vi "Temp_set_statemachine.vi"() -> ()   [LabVIEW 2022 SP3]
uses:
  set_temp_and_time_enum.ctl
  Command_buttons.ctl
  ctl_timer_fgv_states_enum.ctl
  Written_command.ctl
  Prog_time_control.ctl
panel:
  in  "stop":bool
  in  "Temp1 reached? 2":bool
  in  "Temp1 reached?":bool
  out "Written command":T1
  in  "Temperature-time\nprogram":T2
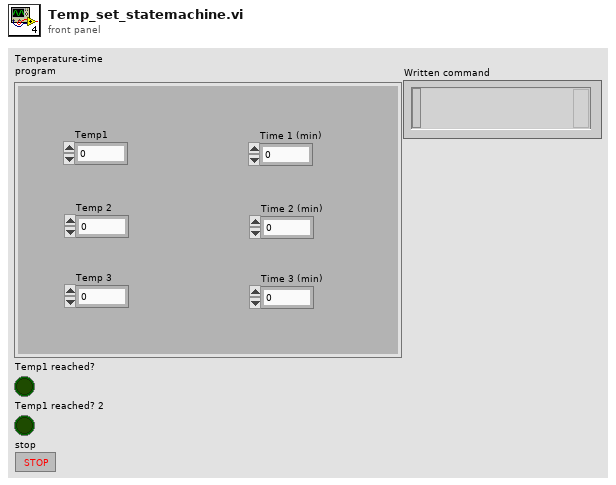
[diagram p1: front panel]
types:
  T1 = typedef "Written_command.ctl" = string
  T2 = typedef "Prog_time_control.ctl" = cluster{"Temp1":dbl, "Temp 2":dbl, "Temp 3":dbl, "Time 1 (min)":dbl, "Time 2 (min)":dbl, "Time 3 (min)":dbl}
  T3 = typedef "set_temp_and_time_enum.ctl" = enum16{"Init", "Set temp1", "Temp1 reached", "Set temp 2", "Temp2 reached", "Set temp 3", "Temp3 reached", "End"}
  T4 = typedef "ctl_timer_fgv_states_enum.ctl" = enum16{"RESET", "GET"}
  T5 = typedef "Command_buttons.ctl" = enum32{"P0", "P1", "F?", "S?", "Sn", "UC", "UF"}
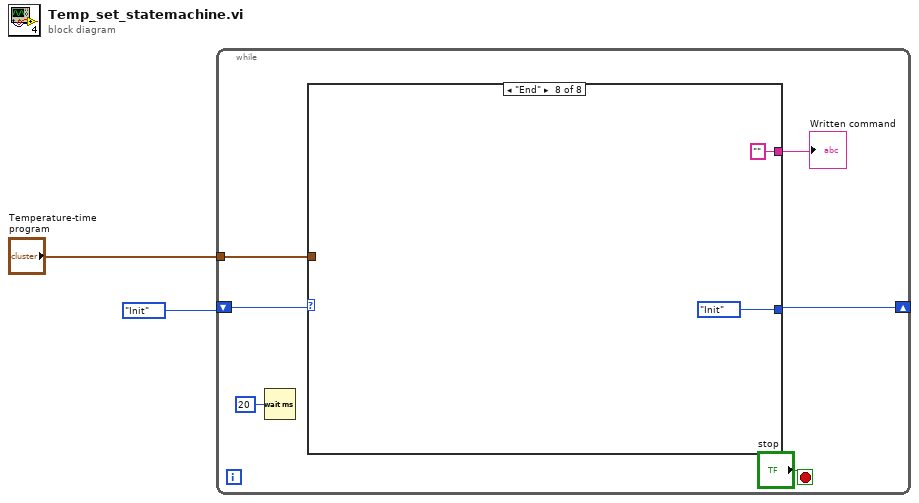
[diagram p0: block diagram]
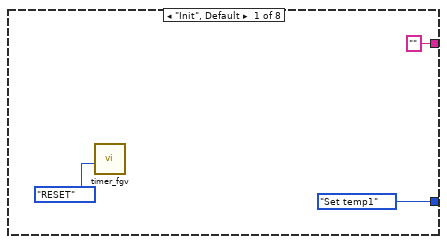
[diagram p2: hidden frame]
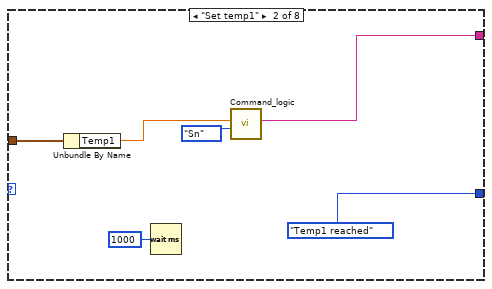
[diagram p3: hidden frame]
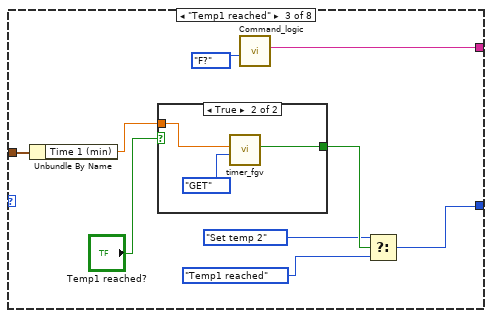
[diagram p4: hidden frame]
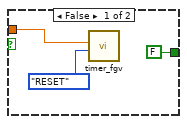
[diagram p5: hidden frame]
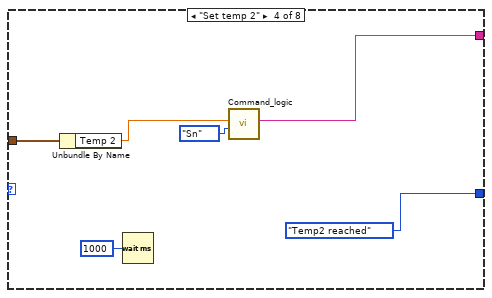
[diagram p6: hidden frame]
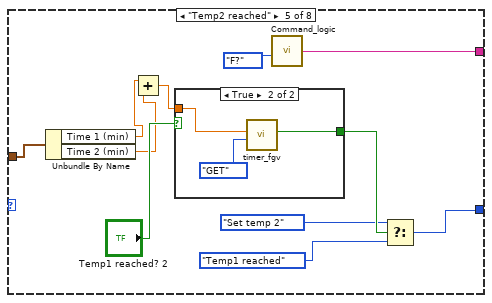
[diagram p7: hidden frame]
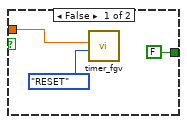
[diagram p8: hidden frame]
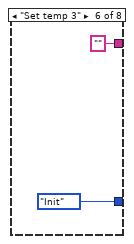
[diagram p9: hidden frame]
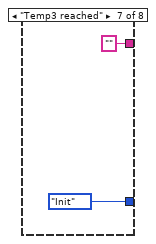
[diagram p10: hidden frame]
diagram:
  n1 = while {
    tunnel: "Temperature-time\nprogram" -> [w8]
    shift-right: [w7] -> _
    shift-left: set_temp_and_time_enum."Init" ("Enum") -> [w6]
    stop <- "stop" stop-if-true
    n2 = Wait (ms)(milliseconds to wait=u32 20) -> ()  [unwired: 1 out]
    n3 = case shown="\"End\"" w6 {
      tunnel: w8 -> [_ w16 w25 w37 w45 _ _ _]
      tunnel: [T1 "" ("Written command") w14 w18 w35 w40 T1 "" ("Written command") T1 "" ("Written command") T1 "" ("Written command")] -> w3
      tunnel: [set_temp_and_time_enum."Set temp1" ("Enum") set_temp_and_time_enum."Temp1 reached" ("Enum") w20 set_temp_and_time_enum."Temp2 reached" ("Enum") w39 set_temp_and_time_enum."Init" ("Enum") set_temp_and_time_enum."Init" ("Enum") set_temp_and_time_enum."Init" ("Enum")] -> w7
      frame "Init", Default {
        n4 = call "timer_fgv.vi"("Operation"=ctl_timer_fgv_states_enum."RESET") -> ()  [unwired: 10 in, 1 out]
      }
      frame "Set temp1" {
        n5 = Unbundle By Name(w16) -> ("Temp1"=w15:dbl)
        n6 = Wait (ms)(milliseconds to wait=u32 1000) -> ()  [unwired: 1 out]
        n7 = call "Command_logic.vi"("Command Radio Buttons"=Command_buttons."Sn", "Temperature\nto set"=w15) -> ("Written command"=w14:T1)  [unwired: 9 in]
      }
      frame "Temp1 reached" {
        n8 = Unbundle By Name(w25) -> ("Time 1 (min)"=w24:dbl)
        n9 = case shown="True" "Temp1 reached?" {
          tunnel: w24 -> [w28 w32]
          tunnel: [FALSE ("TIme passed?") w30] -> w23
          frame False {
            n10 = call "timer_fgv.vi"("Operation"=ctl_timer_fgv_states_enum."RESET", "TImer"=w28) -> ()  [unwired: 9 in, 1 out]
          }
          frame True {
            n11 = call "timer_fgv.vi"("Operation"=ctl_timer_fgv_states_enum."GET", "TImer"=w32) -> ("TIme passed?"=w30:bool)  [unwired: 9 in]
          }
        }
        n12 = call "Command_logic.vi"("Command Radio Buttons"=Command_buttons."F?") -> ("Written command"=w18:T1)  [unwired: 10 in]
        n13 = Select(t=set_temp_and_time_enum."Set temp 2" ("Enum"), s=w23, f=set_temp_and_time_enum."Temp1 reached" ("Enum")) -> (s? t:f=w20:T3)
      }
      frame "Set temp 2" {
        n14 = Unbundle By Name(w37) -> ("Temp 2"=w36:dbl)
        n15 = Wait (ms)(milliseconds to wait=u32 1000) -> ()  [unwired: 1 out]
        n16 = call "Command_logic.vi"("Command Radio Buttons"=Command_buttons."Sn", "Temperature\nto set"=w36) -> ("Written command"=w35:T1)  [unwired: 9 in]
      }
      frame "Temp2 reached" {
        n17 = Unbundle By Name(w45) -> ("Time 1 (min)"=w43:dbl, "Time 2 (min)"=w42:dbl)
        n18 = Add(x=w43, y=w42) -> (x+y=w44:dbl)
        n19 = case shown="True" "Temp1 reached? 2" {
          tunnel: w44 -> [w51 w55]
          tunnel: [FALSE ("TIme passed?") w53] -> w48
          frame False {
            n20 = call "timer_fgv.vi"("Operation"=ctl_timer_fgv_states_enum."RESET", "TImer"=w51) -> ()  [unwired: 9 in, 1 out]
          }
          frame True {
            n21 = call "timer_fgv.vi"("Operation"=ctl_timer_fgv_states_enum."GET", "TImer"=w55) -> ("TIme passed?"=w53:bool)  [unwired: 9 in]
          }
        }
        n22 = call "Command_logic.vi"("Command Radio Buttons"=Command_buttons."F?") -> ("Written command"=w40:T1)  [unwired: 10 in]
        n23 = Select(t=set_temp_and_time_enum."Set temp 2" ("Enum"), s=w48, f=set_temp_and_time_enum."Temp1 reached" ("Enum")) -> (s? t:f=w39:T3)
      }
      frame "Set temp 3" {
      }
      frame "Temp3 reached" {
      }
      frame "End" {
      }
    }
    "Written command" <- w3
  }
